vi "CRUD Testbed.vi"() -> ()   [LabVIEW 2020]
uses:
  AlbumMap/AlbumMap.lvclass
  C:/Program Files/National Instruments/LabVIEW 2020/vi.lib/Viviota/shared/ORM.lvlibp/ORM/TypeMap/TypeMap.lvclass
  Album/Album.lvclass
  Album/Album.lvclass/Album.ctl
  Album/Write Primary Key.vi
  Album/Write Title.vi
  fe3253a3-969b-4c29-9f6b-b8ef4fddbfd0.vi
  95b3caf8-fdfb-4d65-b9ce-178ac661f7ba.vi
  0f7b7644-e09b-4925-812c-9c56f05cb0c9.vi
  5ec95696-ccc5-4566-a2f5-ed917608f8a3.vi
  Album/Read Primary Key.vi
  Album/Read Title.vi
  fe3253a3-969b-4c29-9f6b-b8ef4fddbfd0.vi/35b31214-e0d6-4ae0-b34c-13eba9df70db.vi
  fe3253a3-969b-4c29-9f6b-b8ef4fddbfd0.vi/2e8f1eab-5a58-47e6-9224-d0a2895e31fd.vi
  95b3caf8-fdfb-4d65-b9ce-178ac661f7ba.vi/ce8babb2-619c-4b95-b634-e027cd54a13e.vi
  95b3caf8-fdfb-4d65-b9ce-178ac661f7ba.vi/383c36e0-7191-4c70-923d-4cc1411f3794.vi
  95b3caf8-fdfb-4d65-b9ce-178ac661f7ba.vi/dcffdf9a-60b2-440f-af14-9d618c05381d.vi
  0f7b7644-e09b-4925-812c-9c56f05cb0c9.vi/bf74eca6-e633-4dc5-891a-edef426d4fd9.vi
  5ec95696-ccc5-4566-a2f5-ed917608f8a3.vi/93c2cd5d-a53a-4cc2-b8c3-9c3eef6598b6.vi
  <vilib>/Viviota/shared/ORM.lvlibp/ORM/TypeMap/Write Table Name.vi
  <vilib>/Viviota/shared/ORM_DBC_Mssql.lvlibp/SQL Connect.vi
  <vilib>/Utility/error.llb/Error Cluster From Error Code.vi
  <vilib>/Viviota/shared/ORM.lvlibp/ORM/TypeMap/Read TypeMap.vi
  <vilib>/Viviota/shared/ORM.lvlibp/ORM/SqlMapper/End Transaction.vi
  <vilib>/Viviota/shared/ORM.lvlibp/ORM/TypeMap/TypeMap.lvclass
  <vilib>/Viviota/shared/ORM.lvlibp/ORM/SqlMapper/SqlMapper.lvclass
  ORM_API/ORM_API.lvlib
  <vilib>/Viviota/shared/ORM_DBC_Mssql.lvlibp/DBC.lvclass
panel:
  out "affectedRows":i32
  out "output cluster":cluster{"Primary Key":i64, "Title":string}
  out "error out":errorcluster
  in  "Enum":enum16{"Create", "Read", "Update", "Destroy"}(ring)
  in  "input cluster":cluster{"Primary Key":i64, "Title":string}
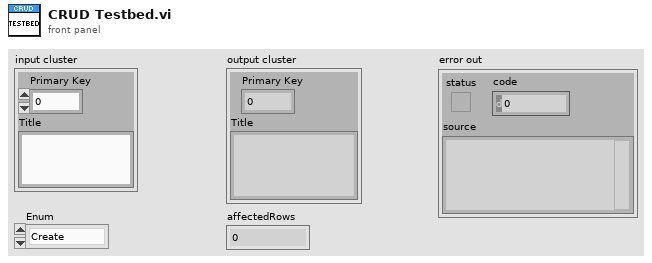
[diagram p1: front panel]
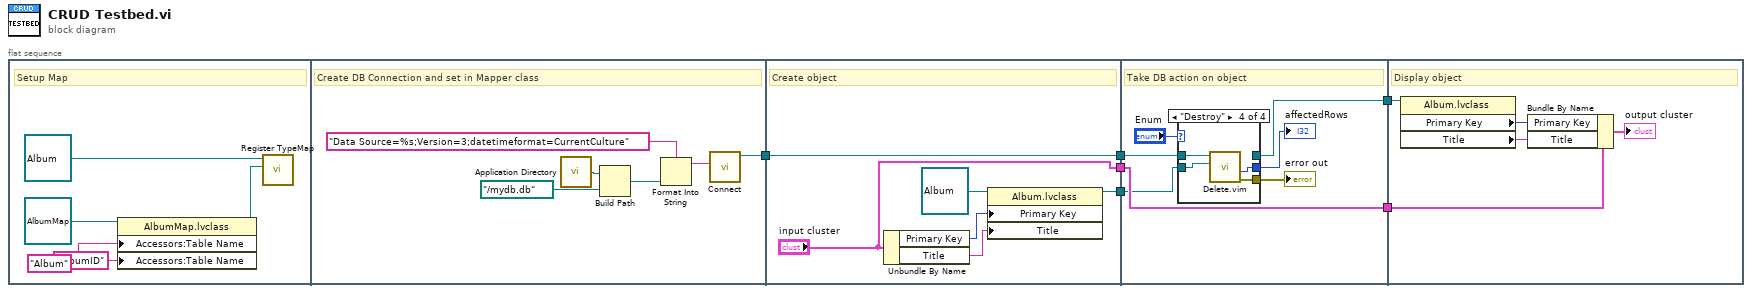
[diagram p0: block diagram]
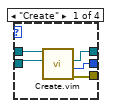
[diagram p2: hidden frame]
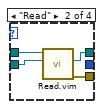
[diagram p3: hidden frame]
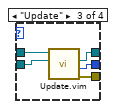
[diagram p4: hidden frame]
diagram:
  n1 = flat-sequence {
    tunnel: [w12] -> w6
    tunnel: w6 -> [w18]
    tunnel: ["input cluster"] -> w5
    tunnel: [w19] -> w4
    tunnel: [w18] -> w3
    tunnel: w5 -> [w27]
    tunnel: w4 -> [w24]
    tunnel: w3 -> [w28]
    tunnel: [w27] -> w2
    tunnel: [w26] -> w1
    tunnel: w2 -> [w50]
    tunnel: w1 -> [w49]
    frame #0 {
      # "Setup Map"
      n2 = property class="AlbumMap.lvclass"(reference=refnum<class "AlbumMap.lvclass"> refnum ("AlbumMap.lvclass"), "Accessors:Table Name"="Album" ("Log Table Name"), "Accessors:Table Name"="AlbumID" ("Table Name")) -> (reference out=w9:refnum<class "AlbumMap.lvclass">)  [unwired: 1 in, 1 out]
      n3 = call <vilib>:"Register TypeMap.vi"("TypeMap in"=w9, "object in"=refnum<class "Album.lvclass"> refnum ("Album.lvclass")) -> ()  [unwired: 7 in, 3 out]
    }
    frame #1 {
      # "Create DB Connection and set in Mapper class"
      n4 = call <vilib>:"Application Directory.vi"() -> ("Application Directory"=w16:path)
      n5 = Build Path(base path=w16, name or relative path=path "../mydb.db" ("file out")) -> (appended path=w17:path)
      n6 = Format Into String(format string="Data Source=%s;Version=3;datetimeformat=CurrentCulture" ("connectionStringName"), w17) -> (resulting string=w13:string)  [unwired: 2 in, 1 out]
      n7 = call-poly "Connect.vi"("Connection String"=w13) -> ("SQL Mapper"=w12:refnum<class "SqlMapper.lvclass">)  [unwired: 9 in, 1 out]
    }
    frame #2 {
      # "Create object"
      n8 = Unbundle By Name("input cluster") -> ("Primary Key"=w21:i64, "Title"=w22:string)
      n9 = property class="Album.lvclass"(reference=refnum<class "Album.lvclass"> refnum, "Primary Key"=w21, "Title"=w22) -> (reference out=w19:refnum<class "Album.lvclass">)  [unwired: 1 in, 1 out]
    }
    frame #3 {
      # "Take DB action on object"
      n10 = case shown="\"Destroy\"" "Enum" {
        tunnel: w24 -> [w34 w36 w40 w47]
        tunnel: w28 -> [w35 w39 w44 w48]
        tunnel: [w33 w38 w43 _] -> w26
        tunnel: [w31 w37 w41 w46] -> w30
        tunnel: [w32 _ w42 w45] -> w25
        frame "Create" {
          n11 = call "Create.vim"("object in"=w34, "SqlMapper in"=w35) -> ("error out"=w31:errorcluster, "id"=w32:i32, "object out"=w33:refnum<class "Album.lvclass">)  [unwired: 6 in, 1 out]
        }
        frame "Read" {
          n12 = call "Read.vim"("object in"=w36, "SqlMapper in"=w39) -> ("error out"=w37:errorcluster, "object out"=w38:refnum<class "Album.lvclass">)  [unwired: 6 in, 2 out]
        }
        frame "Update" {
          n13 = call "Update.vim"("object in"=w40, "SqlMapper in"=w44) -> ("error out"=w41:errorcluster, "affectedRows"=w42:i32, "object out"=w43:refnum<class "Album.lvclass">)  [unwired: 6 in, 1 out]
        }
        frame "Destroy" {
          n14 = call "Delete.vim"("object in"=w47, "SqlMapper in"=w48) -> ("error out"=w46:errorcluster, "affectedRows"=w45:i32)  [unwired: 7 in, 1 out]
        }
      }
      "error out" <- w30
      "affectedRows" <- w25
    }
    frame #4 {
      # "Display object"
      n15 = property class="Album.lvclass"(reference=w49) -> ("Primary Key"=w53:i64, "Title"=w52:string)  [unwired: 1 in, 2 out]
      n16 = Bundle By Name(cluster=w50, "Primary Key"=w53, "Title"=w52) -> (→"output cluster":cluster{"Primary Key":i64, "Title":string})
    }
  }
